vi "DAQ_read_T_dT.vi"(8 "error in (no error)":errorcluster, 11 "Refnum in":refnum<k21>) -> (0 "error out":errorcluster, 2 "data":dbl[](array[numeric]) format="%0.2f", 3 "Refnum out":refnum<k21>)   [LabVIEW 2021, in "DAQ_Termopares.lvlib"]
uses:
  DAQ_Termopares.lvlib
  <vilib>/DAQmx/read.llb/DAQmx Read (Analog 1D DBL NChan 1Samp).vi
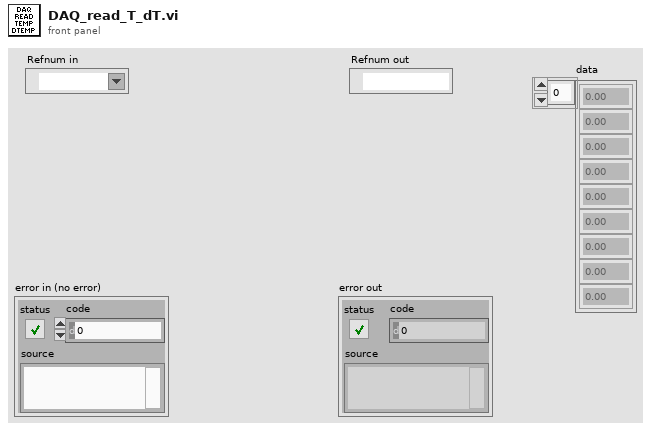
[diagram p1: front panel]
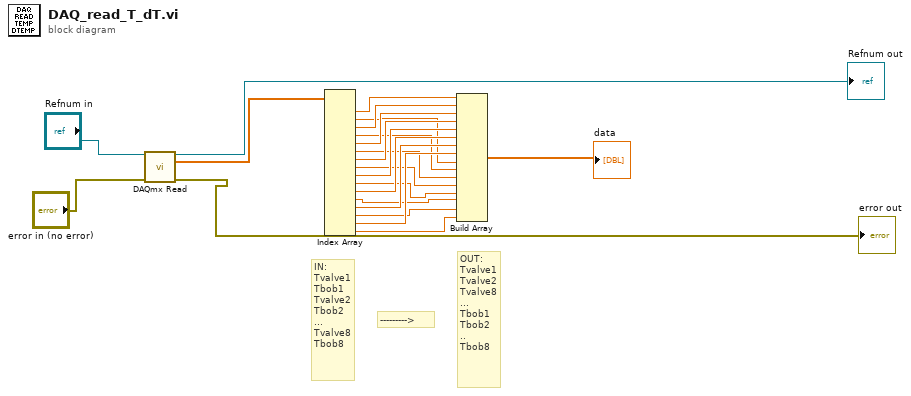
[diagram p0: block diagram]
diagram:
  # "OUT:\nTvalve1\nTvalve2\nTvalve8\n...\nTbob1\nTbob2\n..\nTbob8"
  # "--------->"
  # "IN:\nTvalve1\nTbob1\nTvalve2\nTbob2\n...\nTvalve8\nTbob8"
  n1 = call-poly <vilib>:"DAQmx Read.vi"("task/channels in"="Refnum in", "error in"="error in (no error)") -> ("task out"=→"Refnum out":refnum<k21>, "data"=w18:dbl[], "error out"=→"error out":errorcluster)  [unwired: 11 in]
  n2 = Index Array(array=w18) -> (element #1=w17:dbl, element #2=w9:dbl, element #3=w16:dbl, element #4=w8:dbl, element #5=w15:dbl, element #6=w7:dbl, element #7=w14:dbl, element #8=w6:dbl, element #9=w13:dbl, element #10=w5:dbl, element #11=w12:dbl, element #12=w4:dbl, element #13=w11:dbl, element #14=w3:dbl, element #15=w10:dbl, element #16=w2:dbl)  [unwired: 16 in]
  n3 = Build Array(w17, w16, w15, w14, w13, w12, w11, w10, w9, w8, w7, w6, w5, w4, w3, w2) -> (→"data":dbl[])
